vi "FdxCmdTxModeControlCvi.vi"(8 "error in":errorcluster, 9 "RerosPortDelay":u32, 10 "TransmitMode":u32(ring) items=["FDX_TX_GENERIC", "FDX_TX_REPLAY", "FDX_TX_INDIVIDUAL"], 11 "InstrumentHandle_port":u32) -> (0 "error out":errorcluster, 3 "InstrumentHandle_port":u32)   [LabVIEW 2020, in "AIM664LV.lvlib"]
doc: "This function is used to configure the operational mode of the transmit port."
uses:
  AIM664LV.lvlib
  AFDX_LibraryAdmin/FdxGlobalDllPath.vi
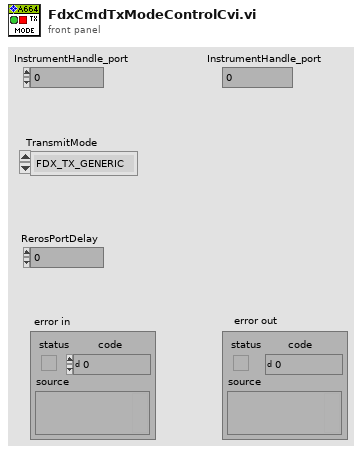
[diagram p1: front panel]
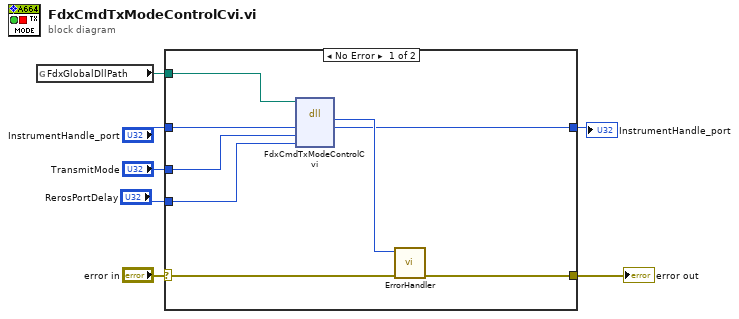
[diagram p0: block diagram]
diagram:
  n1 = global read "FdxGlobalDllPath.vi" "FdxGlobalDllPath"() -> (w5:path)
  n2 = case shown="No Error" "error in" {
    selector: "error in" -> [w14 w17]
    tunnel: [w15 w17] -> w7
    tunnel: w5 -> [w12 _]
    tunnel: [w11 w16] -> w4
    tunnel: "InstrumentHandle_port" -> [w10 w16]
    tunnel: "RerosPortDelay" -> [w9 _]
    tunnel: "TransmitMode" -> [w8 _]
    frame No Error {
      n3 = dll-call lib="aim_fdx.19.dll" fn="FdxCmdTxModeControlCvi"(path in=w12, "InstrumentHandle"=w10, "TransmitMode"=w8, "RerosPortDelay"=w9) -> ("status"=w13:i32, "InstrumentHandle"=w11:u32)  [unwired: 4 in, 2 out]
      n4 = call "ErrorHandler.vi"("error in"=w14, "AIM Error"=w13) -> ("error out"=w15:errorcluster)  [unwired: 9 in]
    }
    frame Error {
    }
  }
  "error out" <- w7
  "InstrumentHandle_port" <- w4
